vi "User Get By Email.vi"(8 "error in (no error)":errorcluster, 10 "Email Address (\"\")":string, 11 "Connection Refnum":T1) -> (0 "error out":errorcluster, 2 "User":T2, 3 "Connection Refnum":T1, 4 "Data Present?":bool)   [LabVIEW 2011]
uses:
  User Record.ctl
  SI.LIB/ODBC/SQL Controls/Connection Refnum.ctl
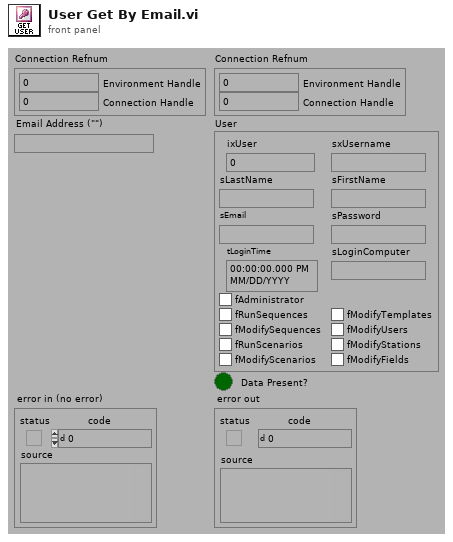
[diagram p1: front panel]
types:
  T1 = typedef "Connection Refnum.ctl" = cluster{"Environment Handle":i32, "Connection Handle":i32}
  T2 = typedef "User Record.ctl" = cluster{"ixUser":i32, "sxUsername":string, "sLastName":string, "sFirstName":string, "sEmail":string, "sPassword":string, "tLoginTime":timestamp, "sLoginComputer":string, "fAdministrator":bool, "fRunSequences":bool, "fModifySequences":bool, "fRunScenarios":bool, "fModifyScenarios":bool, "fModifyTemplates":bool, "fModifyUsers":bool, "fModifyStations":bool, "fModifyFields":bool}
  T3 = typedef "Statement Refnum.ctl" = cluster{"Statement Handle":i32, "Parameter Number":u16}
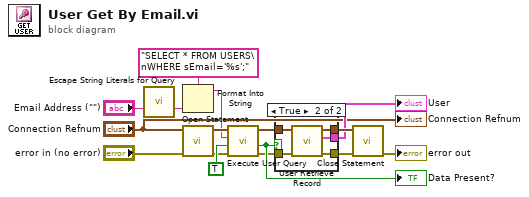
[diagram p0: block diagram]
diagram:
  n1 = call "Escape String Literals for Query.vi"("String"="Email Address (\"\")") -> ("escaped String"=w5:string)  [unwired: 1 in, 13 out]
  n2 = Format Into String(format string="SELECT * FROM USERS\nWHERE sEmail='%s';" ("User Query"), w5) -> (resulting string=w7:string)  [unwired: 2 in, 1 out]
  n3 = call "Open Statement.vi"("error in (no error)"="error in (no error)", "Connection Refnum"="Connection Refnum") -> ("error out"=w8:errorcluster, "Statement Refnum"=w9:T3)  [unwired: 4 out]
  n4 = call "Execute User Query.vi"("error in (no error)"=w8, "Return Data? (f)"=TRUE, "User Query"=w7, "Statement Refnum"=w9) -> ("error out"=w15:errorcluster, "Data Present?"=w16:bool, "Statement Refnum"=w14:T3)  [unwired: 1 out]
  "Data Present?" <- w16
  n5 = case shown="True" w16 {
    tunnel: w15 -> [w17 w23]
    tunnel: w14 -> [w18 w22]
    tunnel: [w17 w20] -> w11
    tunnel: [w18 w21] -> w12
    tunnel: [_ w19] -> w3
    frame False {
    }
    frame True {
      n6 = call "User Retrieve Record.vi"("error in (no error)"=w23, "Statement Refnum"=w22) -> ("error out"=w20:errorcluster, "User Record"=w19:T2, "Statement Refnum"=w21:T3)  [unwired: 7 out]
    }
  }
  "User" <- w3
  n7 = call "Close Statement.vi"("error in (no error)"=w11, "Statement Refnum"=w12) -> ("error out"=→"error out":errorcluster)  [unwired: 5 out]
  "Connection Refnum" <- "Connection Refnum"
